vi "002Project.vi"() -> ()   [LabVIEW 2024]
uses:
  Control 3.ctl
  Documents/LabView Projects/Control 1.ctl
  Control 2_1.ctl
  <vilib>/numeric/Random Number (Range) U64.vi
  <vilib>/numeric/sub_Random U32.vi
panel:
  in  "Silinecek ID":dbl
  out "Arama Sonucu":string
  in  "Search":bool
  in  "Remove":bool
  in  "Add":bool
  in  "Stop":bool
  in  "Kullanıcı Bilgileri":T1={"İsim"="", "Yaş"=10.0, "Boy"=1.0} {"Boy" min=1.0 max=2.5 step=0.01; "Yaş" min=10.0 max=100.0}
  out "Kullanıcı Listesi":T2
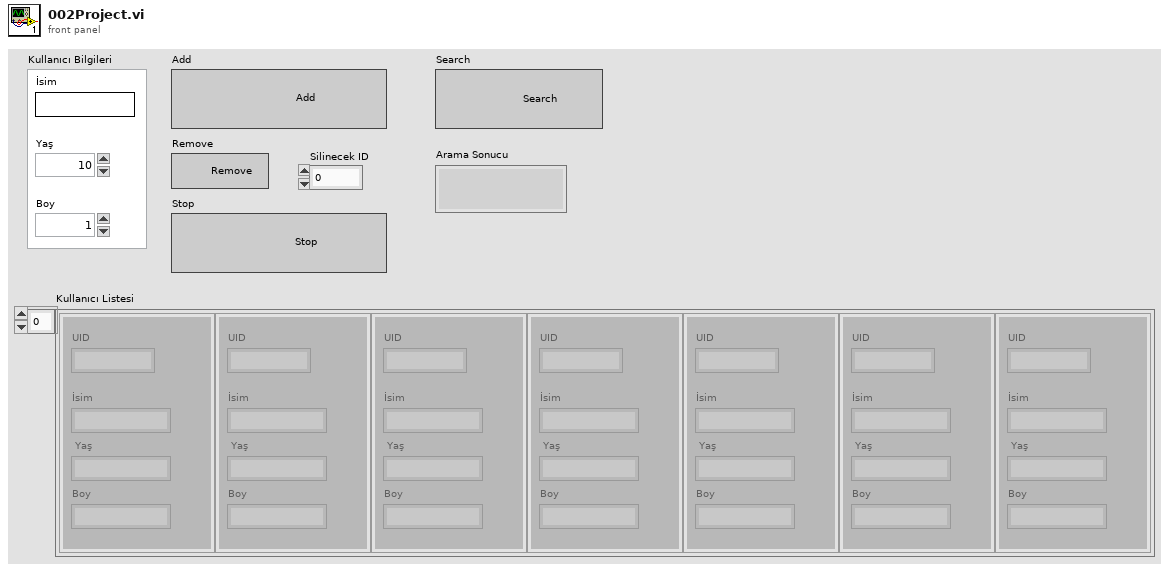
[diagram p1: front panel]
types:
  T1 = typedef "Control 2_1.ctl" = cluster{"İsim":string, "Yaş":dbl, "Boy":dbl}
  T2 = typedef "Control 3.ctl" = T3[]
  T3 = typedef "Control 1.ctl" = cluster{"UID":string, "İsim":string, " Yaş":string, "Boy":string}
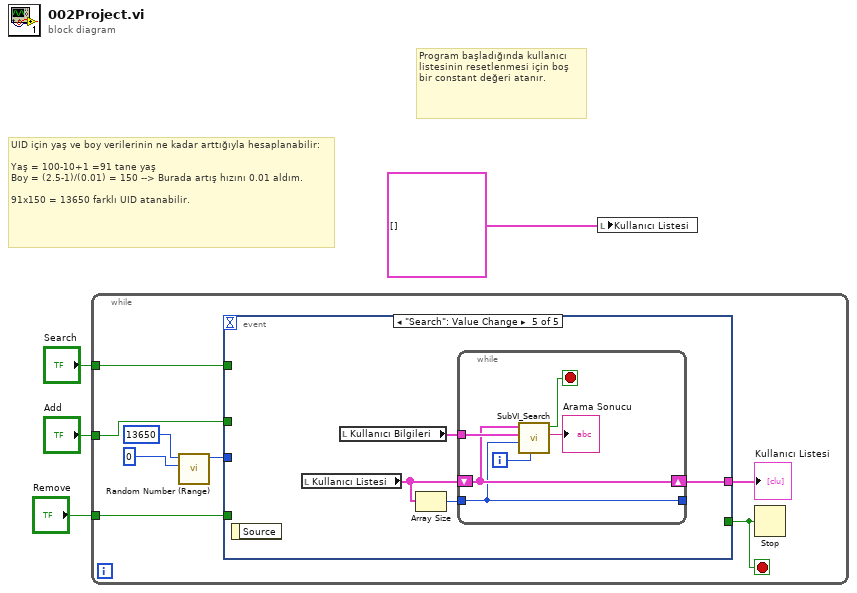
[diagram p0: block diagram]
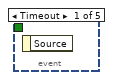
[diagram p2: hidden frame]
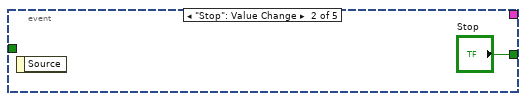
[diagram p3: hidden frame]
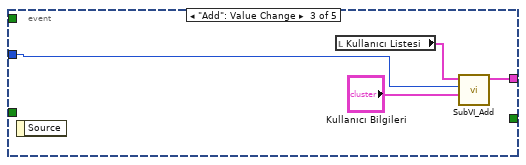
[diagram p4: hidden frame]
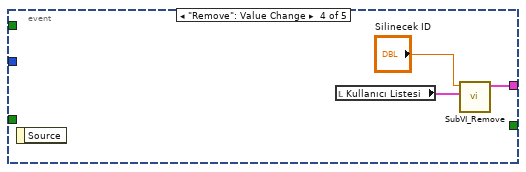
[diagram p5: hidden frame]
diagram:
  # "UID için yaş ve boy verilerinin ne kadar arttığıyla hesaplanabilir:\n\nYaş = 100-10+1 =91 tane yaş \nBoy = (2.5-1)/(0.01) = 150 --> Burada artış hızını 0.01 aldım.\n\n91x150 = 13650 farklı UID atanabilir."
  # "Program başladığında kullanıcı listesinin resetlenmesi için boş bir constant değeri atanır."
  n1 = while {
    tunnel: "Add" -> [w9]
    tunnel: "Search" -> [w6]
    tunnel: "Remove" -> [w7]
    stop <- w5 stop-if-true
    n2 = call-poly <vilib>:"Random Number (Range).vi"("lower bound (0)"=u64 0, "upper bound (100)"=u64 13650) -> ("number"=w10:u64)  [unwired: 9 in]
    n3 = event shown="[4] \"Search\": Value Change" {
      selector: _ -> [_ _ _ _ _]
      dyn-events: _ -> [_ _ _ _ _]
      timeout: _ -> [_ _ _ _ _]
      tunnel: w10 -> [_ _ w14 _ _]
      tunnel: w9 -> [_ _ _ _ _]
      tunnel: [_ _ w17 w18 w23] -> w8
      tunnel: w7 -> [_ _ _ _ _]
      tunnel: w6 -> [_ _ _ _ _]
      tunnel: [_ "Stop" _ _ _] -> w5
      event Timeout {
        n4 = event-data() -> ()  [unwired: 1 in, 1 out]
      }
      event "Stop": Value Change {
        n5 = event-data() -> ()  [unwired: 1 in, 1 out]
      }
      event "Add": Value Change {
        n6 = event-data() -> ()  [unwired: 1 in, 1 out]
        n7 = local read "Kullanıcı Listesi"() -> (w16:T2)
        n8 = call "SubVI_Add.vi"("Kullanıcı Bilgileri"="Kullanıcı Bilgileri", "UID"=w14, "Kullanıcı Listesi in"=w16) -> ("Kullanıcı Listesi out"=w17:T2)  [unwired: 8 in]
      }
      event "Remove": Value Change {
        n9 = event-data() -> ()  [unwired: 1 in, 1 out]
        n10 = local read "Kullanıcı Listesi"() -> (w20:T2)
        n11 = call "SubVI_Remove.vi"("Kullanıcı Listesi in"=w20, "Silinecek ID"="Silinecek ID") -> ("Kullanıcı Listesi out"=w18:T2)  [unwired: 9 in]
      }
      event "Search": Value Change {
        n12 = event-data() -> ()  [unwired: 1 in, 1 out]
        n13 = local read "Kullanıcı Listesi"() -> (w24:T2)
        n14 = local read "Kullanıcı Bilgileri"() -> (w22:T1)
        n15 = Array Size(array=w24) -> (size(s)=w21:i32)
        n16 = while {
          shift-right: [w29] -> w23
          shift-left: w24 -> [w29]
          tunnel: w22 -> [w30]
          tunnel: [w27] -> _
          tunnel: w21 -> [w27]
          i -> [w28]
          stop <- w26 stop-if-true
          n17 = call "SubVI_Search.vi"("Numeric 2"=w28, "Silinecek ID"=w27, "Kullanıcı Bilgileri"=w30, "Kullanıcı Listesi"=w29) -> ("Arama Sonucu"=→"Arama Sonucu":string, "Stop(while)"=w26:bool)  [unwired: 6 in]
        }
      }
    }
    "Kullanıcı Listesi" <- w8
    n18 = Stop(stop? (T)=w5) -> ()
  }
  n19 = local write "Kullanıcı Listesi"(cluster{string, string, string, string}[] []) -> ()
